vi "Wait for Acquisition Complete.vi"(8 "error in (no error)":errorcluster, 9 "Maximum Time (10000 ms)":u32=10000, 11 "VISA resource name":refnum<visa-resource-name>) -> (0 "error out":errorcluster, 3 "VISA resource name out":refnum<visa-resource-name>)   [LabVIEW 2011, in "Agilent DSO1000 Series.lvlib"]
doc: "Waits for the current waveform acquisition to finish. This VI should be called after Initiate VI and before Fetch Waveform VI.\n\n<B>Note:</B> \n\nUse this VI only with other low-level VIs. The high-level VIs automatically incorporate this functionality. This VI does not check the instrument status."
uses:
  <instrlib>/Agilent DSO1000 Series/Agilent DSO1000 Series.lvlib
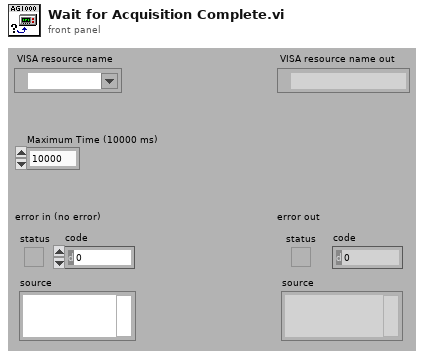
[diagram p1: front panel]
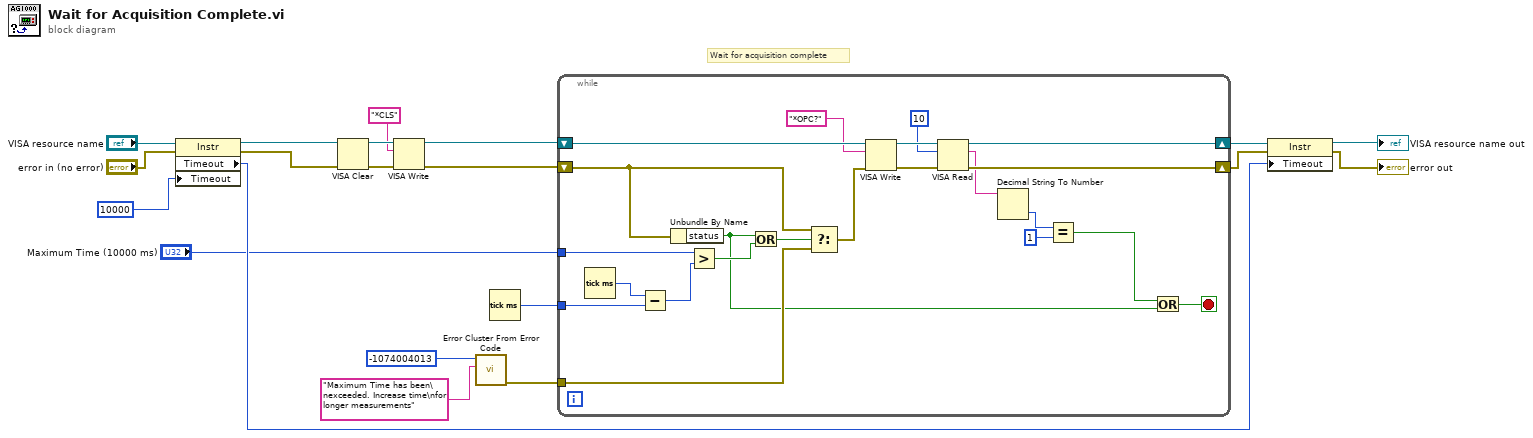
[diagram p0: block diagram]
diagram:
  # "Wait for acquisition complete"
  n1 = property class="Instr"(reference="VISA resource name", error in="error in (no error)", "Timeout"=u32 10000 ("General Settings:Timeout Value")) -> (reference out=w14:refnum<visa-resource-name>, error out=w13:errorcluster, "Timeout"=w8:u32)
  n2 = VISA Clear(VISA resource name=w14, error in (no error)=w13) -> (VISA resource name out=w11:refnum<visa-resource-name>, error out=w12:errorcluster)
  n3 = VISA Write(VISA resource name=w11, write buffer="*CLS", error in (no error)=w12) -> (VISA resource name out=w3:refnum<visa-resource-name>, error out=w2:errorcluster)  [unwired: 1 out]
  n4 = call <vilib>:"Error Cluster From Error Code.vi"("error message (\"\")"="Maximum Time has been\nexceeded. Increase time\nfor longer measurements" ("error message (\"\")"), "error code (0)"=-1074004013) -> ("error out"=w15:errorcluster)  [unwired: 7 in]
  n5 = Tick Count (ms)() -> (millisecond timer value=w20:u32)
  n6 = while {
    tunnel: w20 -> [w41]
    shift-right: [w34] -> w6
    shift-left: w2 -> [w29]
    shift-right: [w35] -> w7
    shift-left: w3 -> [w40]
    tunnel: w15 -> [w30]
    tunnel: "Maximum Time (10000 ms)" -> [w24]
    stop <- w33 stop-if-true
    n7 = Tick Count (ms)() -> (millisecond timer value=w42:u32)
    n8 = Subtract(x=w42, y=w41) -> (x-y=w25:u32)
    n9 = Unbundle By Name(w29) -> ("status"=w27:bool)
    n10 = Greater?(x=w24, y=w25) -> (0:w32:bool)
    n11 = Or(x=w27, y=w32) -> (x .or. y?=w31:bool)
    n12 = Select(t=w29, s=w31, f=w30) -> (s? t:f=w28:errorcluster)
    n13 = VISA Write(VISA resource name=w40, write buffer="*OPC?", error in (no error)=w28) -> (VISA resource name out=w38:refnum<visa-resource-name>, error out=w37:errorcluster)  [unwired: 1 out]
    n14 = VISA Read(VISA resource name=w38, byte count=u32 10, error in (no error)=w37) -> (VISA resource name out=w35:refnum<visa-resource-name>, read buffer=w23:string, error out=w34:errorcluster)  [unwired: 1 out]
    n15 = Decimal String To Number(string=w23) -> (number=w22:i32)  [unwired: 2 in, 1 out]
    n16 = Equal?(x=w22, y=1) -> (x = y?=w26:bool)
    n17 = Or(x=w26, y=w27) -> (x .or. y?=w33:bool)
  }
  n18 = property class="Instr"(reference=w7, error in=w6, "Timeout"=w8) -> (reference out=→"VISA resource name out":refnum<visa-resource-name>, error out=→"error out":errorcluster)
